vi "处理中文字符.vi"(11 "字符":string) -> (3 "标签":string[](array[string]))   [LabVIEW 2018]
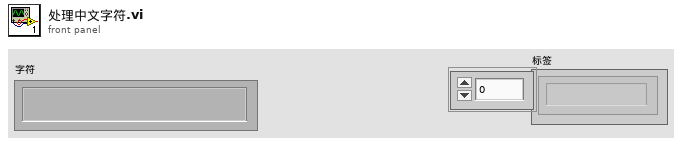
[diagram p1: front panel]
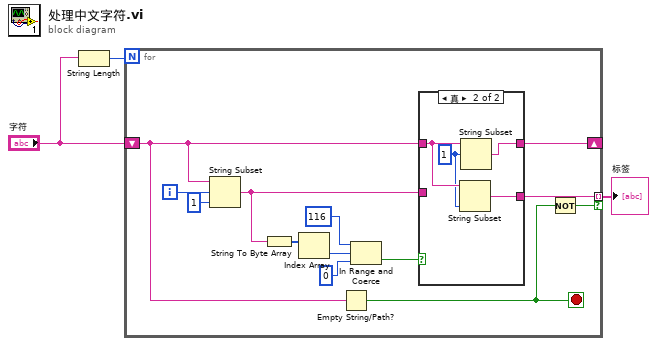
[diagram p0: block diagram]
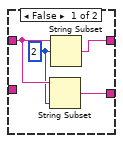
[diagram p2: hidden frame]
diagram:
  n1 = String Length(string="字符") -> (length=w3:i32)
  n2 = for {
    N: w3 -> [_]
    shift-right: [w9] -> _
    shift-left: "字符" -> [w6]
    tunnel: [w7] -> w1 mode=indexing if=w4
    i -> [w16]
    stop <- w5 stop-if-true
    n3 = String Subset(string=w6, offset (0)=w16, length (rest)=1 ("长度（剩余）")) -> (substring=w8:string)
    n4 = String To Byte Array(string=w8) -> (unsigned byte array=w14:u8[])
    n5 = Index Array(array=w14) -> (element=w13:u8)  [unwired: 1 in]
    n6 = Empty String/Path?(string/path=w6) -> (empty?=w5:bool)
    n7 = In Range and Coerce(upper limit=u8 116 ("上限"), x=w13, lower limit=u8 0 ("下限")) -> (In Range?=w10:bool)  [unwired: 1 out]
    n8 = case shown="真" w10 {
      tunnel: w6 -> [w19 w23]
      tunnel: [w20 w24] -> w9
      tunnel: w8 -> [_ _]
      tunnel: [w17 w21] -> w7
      frame False {
        w18 = 2 ("偏移量(0)")
        n9 = String Subset(string=w19, length (rest)=w18) -> (substring=w17:string)  [unwired: 1 in]
        n10 = String Subset(string=w19, offset (0)=w18) -> (substring=w20:string)  [unwired: 1 in]
      }
      frame True {
        w22 = 1 ("偏移量(0)")
        n11 = String Subset(string=w23, length (rest)=w22) -> (substring=w21:string)  [unwired: 1 in]
        n12 = String Subset(string=w23, offset (0)=w22) -> (substring=w24:string)  [unwired: 1 in]
      }
    }
    n13 = Not(x=w5) -> (.not. x?=w4:bool)
  }
  "标签" <- w1
